vi "SW_Shape_Conditions_Array_after_Loading_GZIP.vi"(2 "error in (no error)":errorcluster, 3 "Conditions presets GZipped in":T1) -> (0 "error out":errorcluster, 1 "Conditions presets array out":T3 {"Specifier(s)"."Validity criteria(s)"."Validity value" min=0.0 step=0.1 format="%.2g"; "Specifier(s)"."Value" step=1.0 format="%#.2g"})   [LabVIEW 2018, in "Tracker.lvlib"]
uses:
  Controls/CTL_Conditions_Array.ctl
  Controls/CTL_Conditions_Cluster.ctl
  Controls/CTL_Condition_type.ctl
  Controls/CTL_Comparison_type.ctl
  Controls/CTL_Validity_check_criteria.ctl
  Controls/CTL_Response_info.ctl
  Controls/CTL_Condition_response_type.ctl
  Controls/CTL_Reponse_port_info.ctl
  Controls/CTL_Conditions_All_Presets_Cluster.ctl
  Controls/CTL_Conditions_GZippped_string.ctl
  Tracker.lvlib
panel:
  in  "Condition presets loaded in":T2
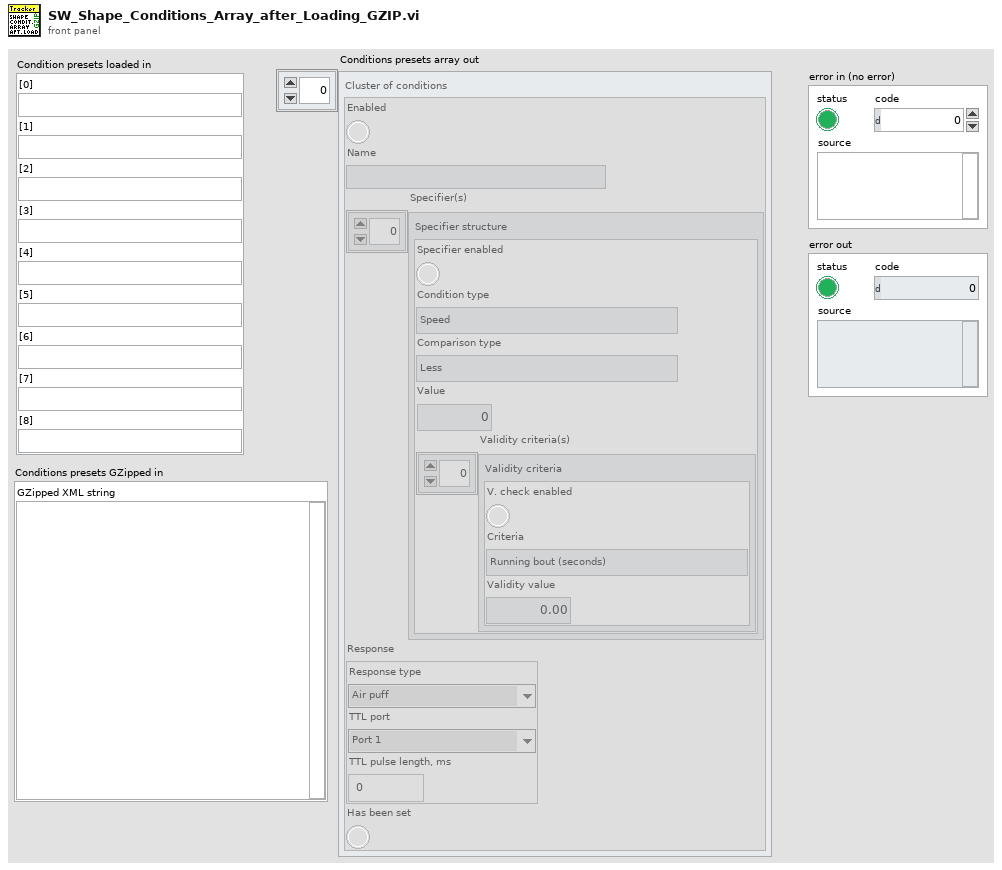
[diagram p1: front panel]
types:
  T1 = typedef "Tracker.lvlib/CTL_Conditions_GZippped_string.ctl" = cluster{"GZipped XML string":string}
  T2 = typedef "Tracker.lvlib/CTL_Conditions_All_Presets_Cluster.ctl" = cluster{"[0]":string, "[1]":string, "[2]":string, "[3]":string, "[4]":string, "[5]":string, "[6]":string, "[7]":string, "[8]":string}
  T3 = typedef "Tracker.lvlib/CTL_Conditions_Array.ctl" = T4[]
  T4 = typedef "Tracker.lvlib/CTL_Conditions_Cluster.ctl" = cluster{"Enabled":bool, "Name":string, "Specifier(s)":cluster{"Specifier enabled":bool, "Condition type":T5, "Comparison type":T6, "Value":dbl, "Validity criteria(s)":cluster{"V. check enabled":bool, "Criteria":T7, "Validity value":dbl}[]}[], "Response":T8, "Has been set":bool}
  T5 = typedef "Tracker.lvlib/CTL_Condition_type.ctl" = enum16{"Speed", "Zone", "Angle to wall"}
  T6 = typedef "Tracker.lvlib/CTL_Comparison_type.ctl" = enum16{"Less", "Less or Equal", "Equal", "Greater or Equal", "Greater", "Not Equal"}
  T7 = typedef "Tracker.lvlib/CTL_Validity_check_criteria.ctl" = enum16{"Running bout (seconds)", "Running bout (meters)"}
  T8 = typedef "Tracker.lvlib/CTL_Response_info.ctl" = cluster{"Response type":T9, "TTL port":T10, "TTL pulse length, ms":dbl}
  T9 = typedef "Tracker.lvlib/CTL_Condition_response_type.ctl" = enum16{"None", "Air puff", "Liquid reward"}
  T10 = typedef "Tracker.lvlib/CTL_Reponse_port_info.ctl" = enum16{"Port 1", "Port 2", "Port 3", "Port 4"}
  T11 = cluster{"Boolean Round":bool, "code":i32, "source":string}
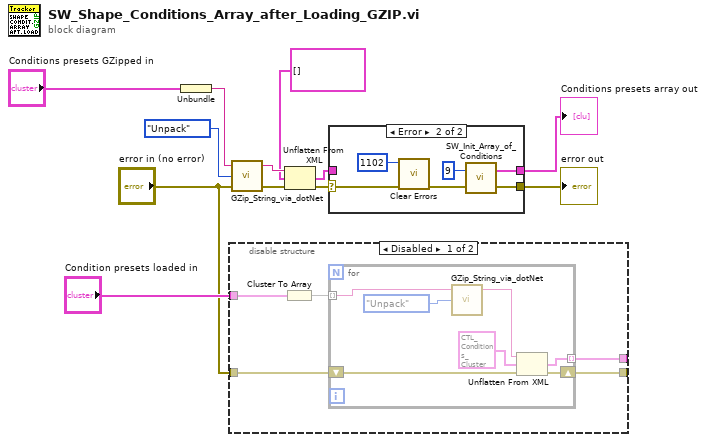
[diagram p0: block diagram]
diagram:
  n1 = Unbundle("Conditions presets GZipped in") -> ("GZipped XML string"=w8:string)
  n2 = disable-structure shown="Disabled" {
    disable-tunnel: "error in (no error)" -> [w17 _]
    disable-tunnel: [w16 _] -> _
    disable-tunnel: [w15 _] -> _
    disable-tunnel: "Condition presets loaded in" -> [w13 _]
    frame Disabled {
      n3 = Cluster To Array(cluster=w13) -> (array=w14:string[])
      n4 = for {
        tunnel: w14 -> [w23] mode=indexing
        tunnel: [w22] -> w15 mode=indexing
        shift-right: [w20] -> w16
        shift-left: w17 -> [w21]
        n5 = call "GZip_String_via_dotNet.vi"("Action"=enum16{"Pack", "Unpack"}."Unpack", "String Input"=w23) -> ("String Output (GZipped/UnGZipped)"=w19:string)  [unwired: 1 in, 2 out]
        n6 = Unflatten From XML(xml string=w19, type=T4 {"Enabled"=FALSE, "Name"="", "Specifier(s)"=[], "Response"={"Response type"=enum."Air puff", "TTL port"=enum."Port 1", "TTL pulse length, ms"=0.0}, "Has been set"=FALSE} ("Cluster of conditions"), error in (no error)=w21) -> (value=w22:T4, error out=w20:errorcluster)
      }
    }
    frame Enabled {
    }
  }
  n7 = call "GZip_String_via_dotNet.vi"("error in (no error)"="error in (no error)", "Action"=enum16{"Pack", "Unpack"}."Unpack", "String Input"=w8) -> ("error out"=w5:errorcluster, "String Output (GZipped/UnGZipped)"=w7:string)  [unwired: 1 out]
  n8 = Unflatten From XML(xml string=w7, type=T3 [] ("Conditions presets array"), error in (no error)=w5) -> (value=w3:T3, error out=w2:errorcluster)
  n9 = case shown="Error" w2 {
    selector: w2 -> [w26 w30]
    tunnel: [w26 w28] -> w12
    tunnel: [w25 w31] -> w11
    tunnel: w3 -> [w25 _]
    frame No Error {
    }
    frame Error {
      n10 = call <vilib>:"Clear Errors.vi"("error in (no error)"=w30, "specific error code to clear (0: all)"=1102) -> ("error out"=w29:errorcluster)  [unwired: 4 in, 1 out]
      n11 = call "SW_Init_Array_of_Conditions.vi"("error in (no error)"=w29, "Array size"=9) -> ("error out"=w28:T11, "Array of conditions"=w31:T3)
    }
  }
  "Conditions presets array out" <- w11
  "error out" <- w12
